vi "fibonacci.vi"() -> ()   [LabVIEW 2018]
panel:
  out "Numeric":dbl
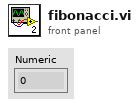
[diagram p1: front panel]
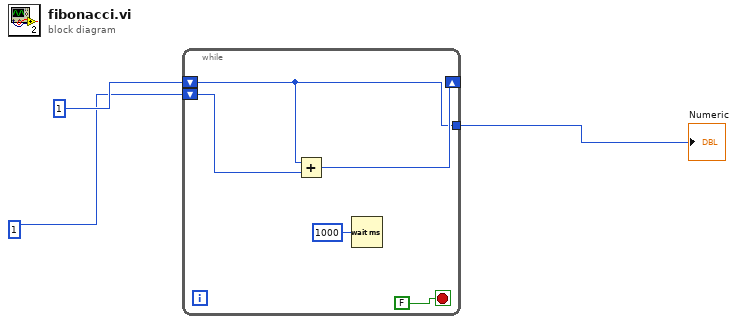
[diagram p0: block diagram]
diagram:
  n1 = while {
    shift-right: [w7] -> _
    shift-left: 1 -> [w6]
    shift-left: 1 -> [w8]
    tunnel: [w6] -> w1
    stop <- FALSE stop-if-true
    n2 = Add(x=w6, y=w8) -> (x+y=w7:i32)
    n3 = Wait (ms)(milliseconds to wait=u32 1000) -> ()  [unwired: 1 out]
  }
  "Numeric" <- w1
